vi "gamma_n__v1.vi"(9 "n":ext, 10 "ƒÀ[n]":ext, 11 "ƒ¿[n]":ext) -> (3 "ƒÁ[n]":ext)   [LabVIEW 2020]
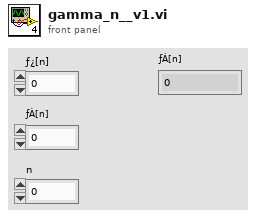
[diagram p1: front panel]
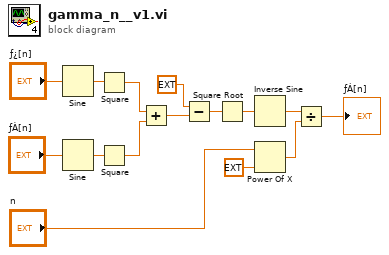
[diagram p0: block diagram]
diagram:
  n1 = Sine(x="ƒ¿[n]") -> (sin(x)=w13:ext)
  n2 = Sine(x="ƒÀ[n]") -> (sin(x)=w12:ext)
  n3 = Square(x=w13) -> (x^2=w10:ext)
  n4 = Square(x=w12) -> (x^2=w9:ext)
  n5 = Add(x=w10, y=w9) -> (x+y=w8:ext)
  n6 = Subtract(x=ext 1.0, y=w8) -> (x-y=w7:ext)
  n7 = Square Root(x=w7) -> (sqrt(x)=w6:ext)
  n8 = Inverse Sine(1:w6) -> (0:w5:ext)
  n9 = Power Of X(1:ext -1.0, 2:"n") -> (0:w2:ext)
  n10 = Divide(x=w5, y=w2) -> (x/y=→"ƒÁ[n]":ext)
